vi "OpenWeb.vi"(8 "error in":errorcluster) -> (0 "error Out":errorcluster caption="error out", 3 "client handle out":T1 caption="客户端句柄输出")   [LabVIEW 2017]
uses:
  <vilib>/httpClient/LabVIEWHTTPClient.lvlib
  <vilib>/httpClient/ClientHandle.ctl
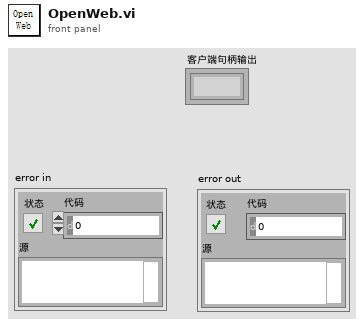
[diagram p1: front panel]
types:
  T1 = typedef "LabVIEWHTTPClient.lvlib/ClientHandle.ctl" = refnum<k1>
  T2 = typedef "HD Config.ctl" = cluster{"ConnectPLC":cluster{"PLC Address":u8[], "PLC Port":i32, "PC Address":u8[]}, "FCO Model 4":cluster{"Com":refnum<visa-resource-name>, "Port":u32}, "FCO Model 7":cluster{"Com":refnum<visa-resource-name>, "Port":u32}, "Flow meter":cluster{"Com":refnum<visa-resource-name>, "Port":u32, "Units":enum16{"Standard", "Volumetric"}}}
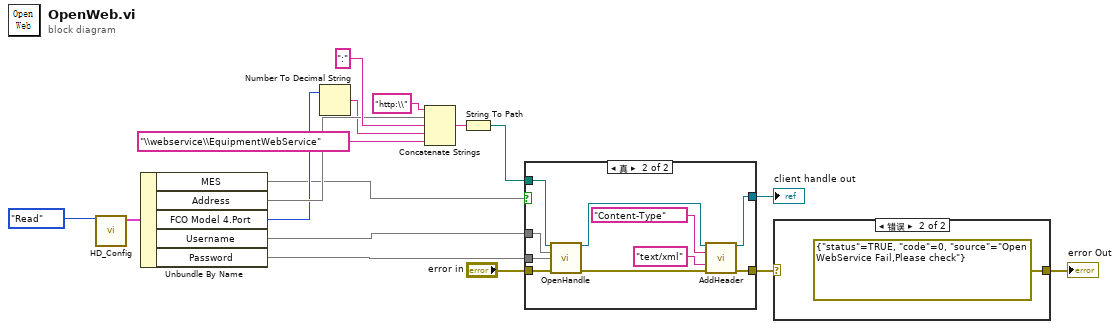
[diagram p0: block diagram]
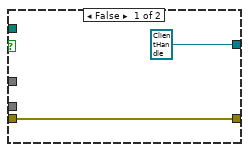
[diagram p2: hidden frame]
diagram:
  n1 = call "HD_Config.vi"("Step"=enum16{"Initial", "Write", "Read"}."Read") -> ("HD Config out"=w2:T2)  [unwired: 9 in, 1 out]
  n2 = Unbundle By Name(w2) -> ("MES"=w1, "Address"=w9, "FCO Model 4.Port"=w8:u32, "Username"=w11, "Password"=w10)
  n3 = Number To Decimal String(number=w8) -> (decimal integer string=w7:string)  [unwired: 1 in]
  n4 = Concatenate Strings("http:\\", w9, ":", w7, "\\webservice\\EquipmentWebService") -> (w13:string)
  n5 = String To Path(string=w13) -> (path=w12:path)
  n6 = case shown="真" w1 {
    tunnel: w12 -> [_ w27]
    tunnel: w11 -> [_ w25]
    tunnel: w10 -> [_ w24]
    tunnel: [T1 refnum ("client handle out") w23] -> w6
    tunnel: "error in" -> [w18 w22]
    tunnel: [w18 w20] -> w4
    frame False {
    }
    frame True {
      n7 = call <vilib>:"OpenHandle.vi"("cookie file"=w27, "username"=w25, "password"=w24, "error in (no error)"=w22) -> ("client handle out"=w28:T1, "error out"=w21:errorcluster)  [unwired: 10 in]
      n8 = call <vilib>:"AddHeader.vi"("client handle"=w28, "header"="Content-Type", "value"="text/xml", "error in (no error)"=w21) -> ("client handle out"=w23:T1, "error out"=w20:errorcluster)  [unwired: 10 in]
    }
  }
  "client handle out" <- w6
  n9 = case shown="错误" w4 {
    selector: w4 -> [w30 _]
    tunnel: [w30 errorcluster {"status"=TRUE, "code"=0, "source"="Open WebService Fail,Please check"} ("error IO")] -> w17
    frame No Error {
    }
    frame Error {
    }
  }
  "error Out" <- w17
